vi "thermometer.vi"(2 "lower  bound":dbl, 4 "upper bound":dbl) -> (0 "Celsius temperature":dbl)   [LabVIEW 2014]
doc: "Randomly output a Celsius temperature value in between the lower and upper bound set with input parameters of lower bound value, and upper bound value."
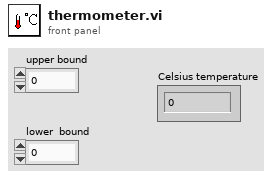
[diagram p1: front panel]
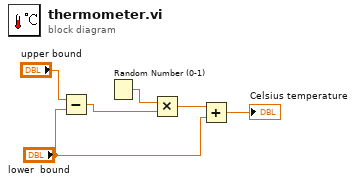
[diagram p0: block diagram]
diagram:
  n1 = Subtract(x="upper bound", y="lower  bound") -> (x-y=w1:dbl)
  n2 = Random Number (0-1)() -> (number: 0 to 1=w6:dbl)
  n3 = Multiply(x=w6, y=w1) -> (x*y=w5:dbl)
  n4 = Add(x=w5, y="lower  bound") -> (x+y=→"Celsius temperature":dbl)
